vi "Downsample image.vi"(8 "error in (no error)":errorcluster, 10 "Original image":u16[][](array[numeric]), 11 "TomoConversion in":refnum<class "TomoConversion.lvclass">) -> (0 "error out":errorcluster, 2 "Downsampled image":u16[][](array[numeric]), 3 "TomoConversion out":refnum<class "TomoConversion.lvclass">)   [LabVIEW 2012, in "TomoConversion.lvclass"]
uses:
  TomoConversion.lvclass
  <vilib>/Analysis/baseanly.llb/Mean (DBL).vi
  <vilib>/Analysis/NI_AALBase.lvlib
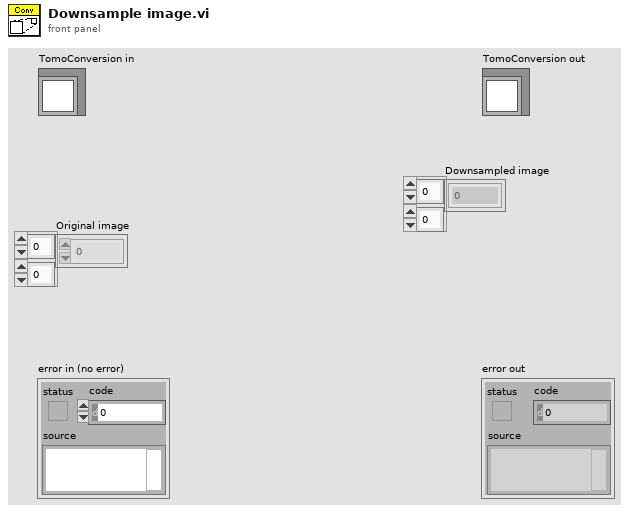
[diagram p1: front panel]
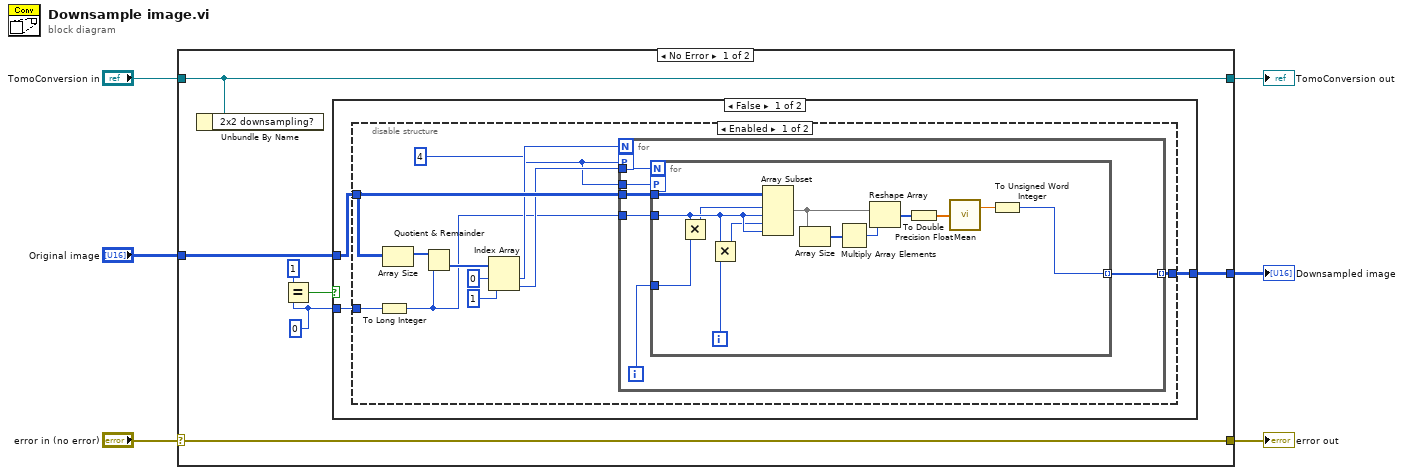
[diagram p0: block diagram]
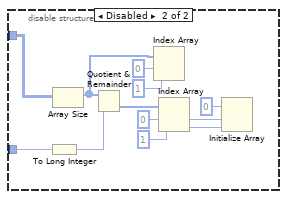
[diagram p2: hidden frame]
diagram:
  n1 = case shown="No Error" "error in (no error)" {
    selector: "error in (no error)" -> [w13 w61]
    tunnel: [w13 w61] -> w5
    tunnel: [w8 w60] -> w3
    tunnel: "TomoConversion in" -> [w8 w60]
    tunnel: "Original image" -> [w12 _]
    tunnel: [w11 _] -> w1
    frame No Error {
      w7 = u32 0 ("y")
      n2 = Unbundle By Name(w8) -> ()  [unwired: 1 out]
      n3 = Equal?(x=u32 1, y=w7) -> (x = y?=w9:bool)
      n4 = case shown="False" w9 {
        tunnel: w7 -> [w16 _]
        tunnel: w12 -> [w15 w59]
        tunnel: [w14 w59] -> w11
        frame False {
          n5 = disable-structure shown="Enabled" {
            disable-tunnel: w16 -> [w26 w51]
            disable-tunnel: w15 -> [w22 w50]
            disable-tunnel: [w18 _] -> w14
            frame Enabled {
              w17 = 4
              n6 = To Long Integer(number=w26) -> (32bit integer=w19:i32)
              n7 = Array Size(array=w22) -> (size(s)=w27:i32[])
              n8 = Quotient & Remainder(x=w27, y=w19) -> (floor(x/y)=w25:i32[])  [unwired: 1 out]
              n9 = Index Array(array=w25, index #1=0 ("index"), index #2=1 ("index")) -> (element #1=w21:i32, element #2=w20:i32)
              n10 = for {
                N: w21 -> [_]
                tunnel: w22 -> [w33]
                tunnel: w20 -> [w31]
                tunnel: w19 -> [w30]
                tunnel: [w29] -> w18 mode=indexing
                workers-P: w17 -> [_]
                tunnel: w17 -> [w28]
                i -> [w32]
                n11 = for {
                  N: w31 -> [_]
                  tunnel: w33 -> [w46]
                  tunnel: w32 -> [w45]
                  tunnel: w30 -> [w44]
                  tunnel: [w34] -> w29 mode=indexing
                  workers-P: w28 -> [_]
                  i -> [w35]
                  n12 = Multiply(x=w44, y=w45) -> (x*y=w43:i32)
                  n13 = Multiply(x=w44, y=w35) -> (x*y=w42:i32)
                  n14 = Array Subset(array=w46, index (row)=w43, length (row)=w44, index (col)=w42, length (col)=w44) -> (w40:u16[][])
                  n15 = Array Size(array=w40) -> (size(s)=w41:i32[])
                  n16 = Multiply Array Elements(1:w41) -> (0:w39:i32)
                  n17 = Reshape Array(w40, w39) -> (w38:u16[])
                  n18 = To Double Precision Float(number=w38) -> (double precision float=w37:dbl[])
                  n19 = call-poly <vilib>:"Mean.vi"("X"=w37) -> ("mean"=w36:dbl)  [unwired: 1 out]
                  n20 = To Unsigned Word Integer(number=w36) -> (unsigned 16bit integer=w34:u16)
                }
              }
            }
            frame Disabled {
              n21 = To Long Integer(number=w51) -> (32bit integer=w52:i32)
              n22 = Array Size(array=w50) -> (size(s)=w47:i32[])
              n23 = Quotient & Remainder(x=w47, y=w52) -> (floor(x/y)=w58:i32[])  [unwired: 1 out]
              n24 = Index Array(array=w47, index #1=0 ("index"), index #2=1 ("index")) -> ()  [unwired: 2 out]
              n25 = Index Array(array=w58, index #1=0 ("index"), index #2=1 ("index")) -> (element #1=w54:i32, element #2=w53:i32)
              n26 = Initialize Array(u16 0 ("element"), w54, w53) -> ()  [unwired: 1 out]
            }
          }
        }
        frame True {
        }
      }
    }
    frame Error {
    }
  }
  "error out" <- w5
  "TomoConversion out" <- w3
  "Downsampled image" <- w1
